vi "Motion Path Planing Sub_VI.vi"(2 "Motion Planning Inputs":T2) -> (5 "No-limit Velocity":dbl, 6 "Motion Profile":T3=enum."Triangular", 7 "Motion Planning Outputs":T1)   [LabVIEW 2017]
uses:
  Motion Type Def.ctl
panel:
  out "total dist":dbl
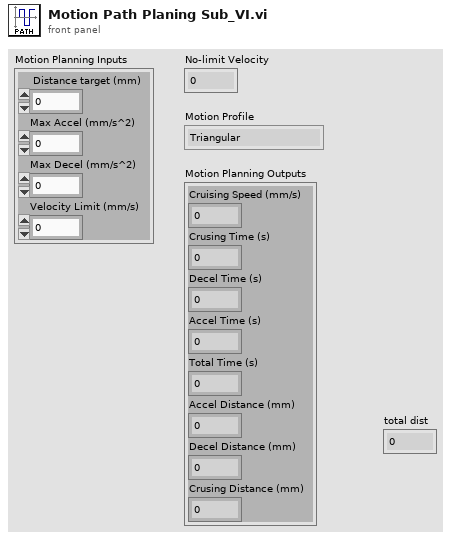
[diagram p1: front panel]
types:
  T1 = cluster{"Cruising Speed (mm/s)":dbl, "Crusing Time (s)":dbl, "Decel Time (s)":dbl, "Accel Time (s)":dbl, "Total Time (s)":dbl, "Accel Distance (mm)":dbl, "Decel Distance (mm)":dbl, "Crusing Distance (mm)":dbl}
  T2 = cluster{" Distance target (mm)":dbl, "Max Accel (mm/s^2)":dbl, "Max Decel (mm/s^2)":dbl, "Velocity Limit (mm/s) ":dbl}
  T3 = typedef "Motion Type Def.ctl" = enum16{"Trapezodial", "Triangular"}
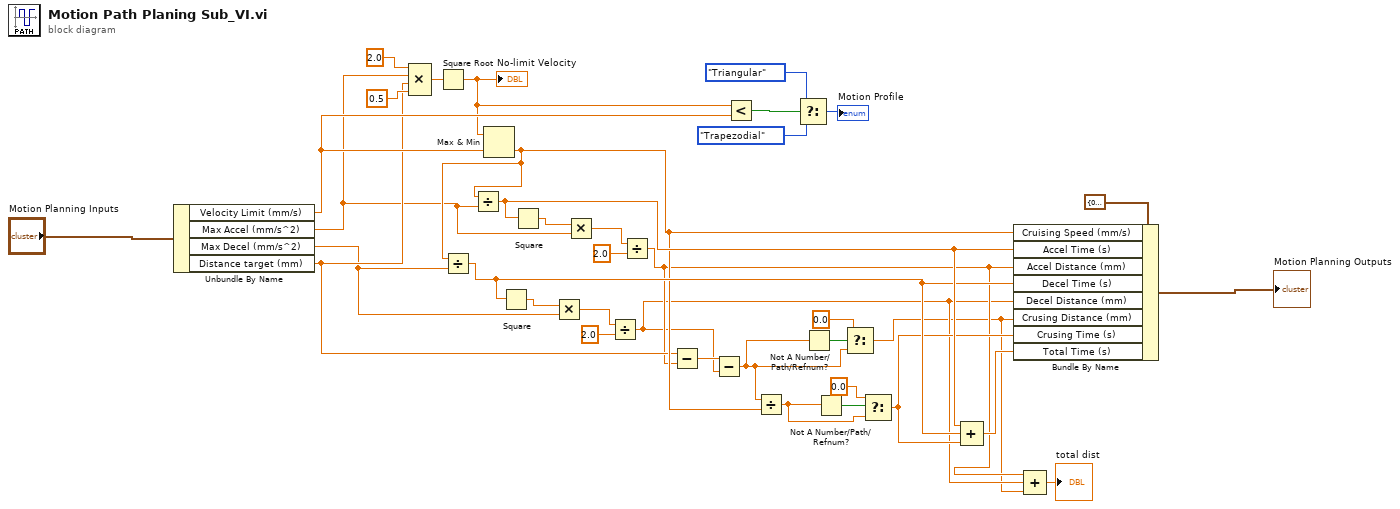
[diagram p0: block diagram]
diagram:
  n1 = Unbundle By Name("Motion Planning Inputs") -> ("Velocity Limit (mm/s)"=w32:dbl, "Max Accel (mm/s^2)"=w24:dbl, "Max Decel (mm/s^2)"=w21:dbl, "Distance target (mm)"=w25:dbl)
  n2 = Compound Arithmetic op=MULTIPLY(2.0 ("value"), w24, w25, 0.5 ("value")) -> (w27:dbl)
  n3 = Square Root(x=w27) -> (sqrt(x)=w31:dbl)
  "No-limit Velocity" <- w31
  n4 = Max & Min(x=w31, y=w32) -> (min(x,y)=w28:dbl)  [unwired: 1 out]
  n5 = Divide(x=w28, y=w21) -> (x/y=w29:dbl)
  n6 = Divide(x=w28, y=w24) -> (x/y=w30:dbl)
  n7 = Square(x=w29) -> (x^2=w18:dbl)
  n8 = Square(x=w30) -> (x^2=w17:dbl)
  n9 = Multiply(x=w18, y=w21) -> (x*y=w19:dbl)
  n10 = Multiply(x=w17, y=w24) -> (x*y=w16:dbl)
  n11 = Divide(x=w19, y=2.0) -> (x/y=w3:dbl)
  n12 = Divide(x=w16, y=2.0) -> (x/y=w4:dbl)
  n13 = Subtract(x=w25, y=w4) -> (x-y=w22:dbl)
  n14 = Subtract(x=w22, y=w3) -> (x-y=w5:dbl)
  n15 = Less?(x=w31, y=w32) -> (x < y?=w33:bool)
  n16 = Divide(x=w5, y=w28) -> (x/y=w11:dbl)
  n17 = Select(t=Motion_Type_Def."Triangular", s=w33, f=Motion_Type_Def."Trapezodial") -> (s? t:f=→"Motion Profile":T3)
  n18 = Not A Number/Path/Refnum?(number/path/refnum=w5) -> (NaN/Path/Refnum?=w8:bool)
  n19 = Not A Number/Path/Refnum?(number/path/refnum=w11) -> (NaN/Path/Refnum?=w12:bool)
  n20 = Select(t=0.0, s=w8, f=w5) -> (s? t:f=w2:dbl)
  n21 = Select(t=0.0, s=w12, f=w11) -> (s? t:f=w10:dbl)
  n22 = Compound Arithmetic op=ADD(w30, w29, w10) -> (w7:dbl)
  n23 = Bundle By Name(cluster=T1 {"Cruising Speed (mm/s)"=0.0, "Crusing Time (s)"=0.0, "Decel Time (s)"=0.0, "Accel Time (s)"=0.0, "Total Time (s)"=0.0, "Accel Distance (mm)"=0.0, "Decel Distance (mm)"=0.0, "Crusing Distance (mm)"=0.0} ("Motion Planning Outputs 2"), "Cruising Speed (mm/s)"=w28, "Accel Time (s)"=w30, "Accel Distance (mm)"=w4, "Decel Time (s)"=w29, "Decel Distance (mm)"=w3, "Crusing Distance (mm)"=w2, "Crusing Time (s)"=w10, "Total Time (s)"=w7) -> (→"Motion Planning Outputs":T1)
  n24 = Compound Arithmetic op=ADD(w4, w3, w2) -> (→"total dist":dbl)
